vi "Timestamp FGV.vi"(7 "Command":T1, 8 "ActualBufferNumber":u32, 10 "ms timer":i32, 11 "Previous frame timestamp":timestamp) -> (2 "Time interval [ms]":i32, 3 "Current frame timestamp":timestamp)   [LabVIEW 2020]
uses:
  Timestamp FGV Command.ctl
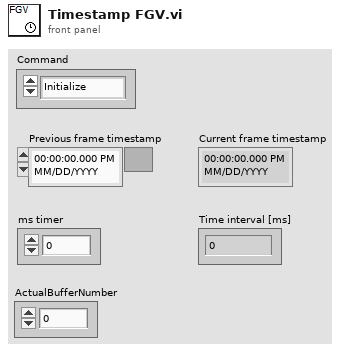
[diagram p1: front panel]
types:
  T1 = typedef "Timestamp FGV Command.ctl" = enum16{"Initialize", "Get"}
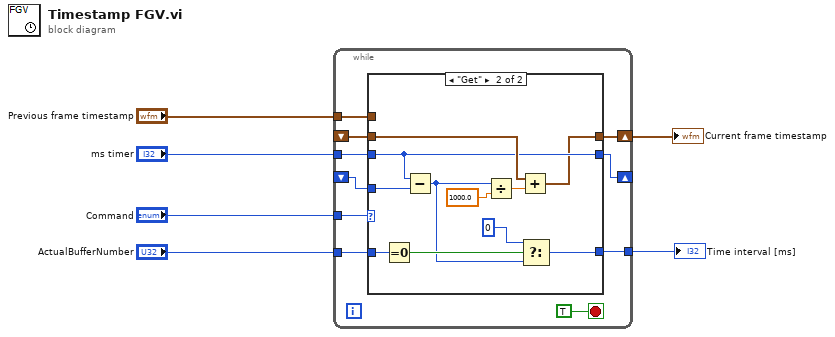
[diagram p0: block diagram]
diagram:
  n1 = while {
    shift-right: [w11] -> w4
    shift-left: _ -> [w8]
    shift-right: [w12] -> _
    shift-left: _ -> [w14]
    tunnel: "Command" -> [w15]
    tunnel: "ms timer" -> [w13]
    tunnel: [w10] -> w3
    tunnel: "ActualBufferNumber" -> [w9]
    tunnel: "Previous frame timestamp" -> [w7]
    stop <- TRUE stop-if-true
    n2 = case shown="\"Get\"" w15 {
      tunnel: w8 -> [_ w27]
      tunnel: w14 -> [_ w26]
      tunnel: w13 -> [w18 w25]
      tunnel: [w18 w25] -> w12
      tunnel: [w17 w24] -> w11
      tunnel: [_ w19] -> w10
      tunnel: w9 -> [_ w22]
      tunnel: w7 -> [w17 _]
      frame "Initialize", Default {
      }
      frame "Get" {
        n3 = Equal To 0?(x=w22) -> (x = 0?=w21:bool)
        n4 = Subtract(x=w25, y=w26) -> (x-y=w20:i32)
        n5 = Divide(x=w20, y=1000.0) -> (x/y=w29:dbl)
        n6 = Add(x=w27, y=w29) -> (x+y=w24:timestamp)
        n7 = Select(t=0, s=w21, f=w20) -> (s? t:f=w19:i32)
      }
    }
  }
  "Time interval [ms]" <- w3
  "Current frame timestamp" <- w4
